vi "dB to Linear.vi"(0 "dB value":dbl format="%.2f", 1 "attenuation?":bool=TRUE) -> (2 "linear value":dbl format="%.2f")   [LabVIEW 2020, in "NI_AAL_Filter.lvlib"]
uses:
  <vilib>/Analysis/NI_AAL_Filter.lvlib
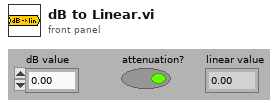
[diagram p1: front panel]
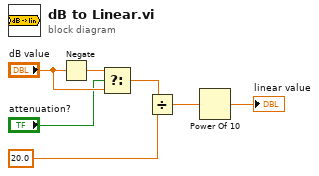
[diagram p0: block diagram]
diagram:
  n1 = Negate(x="dB value") -> (-x=w6:dbl)
  n2 = Select(t=w6, s="attenuation?", f="dB value") -> (s? t:f=w3:dbl)
  n3 = Divide(x=w3, y=20.0) -> (x/y=w2:dbl)
  n4 = Power Of 10(x=w2) -> (10^x=→"linear value":dbl)
